vi "Untitled 1.vi"() -> ()   [LabVIEW 2013]
uses:
  <vilib>/Analysis/6fits.llb/General Linear Fit Algorithm.ctl
  <vilib>/Analysis/NI_AALPro.lvlib
panel:
  in  "algorithm":T1 items=["SVD", "Givens", "Givens2", "Householder", "LU Decomposition", "Cholesky", "SVD for Rank Deficient H"]
  out "residue":dbl
  out "Polynomial Coefficients":dbl[](array[numeric])
  out "Best Polynomial Fit":dbl[](array[numeric])
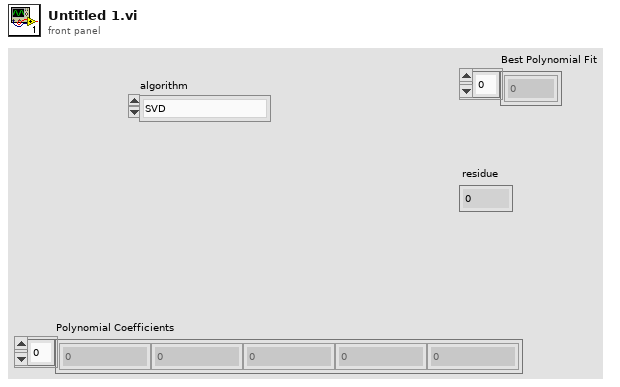
[diagram p1: front panel]
types:
  T1 = typedef "NI_AALPro.lvlib/General Linear Fit Algorithm.ctl" = u16
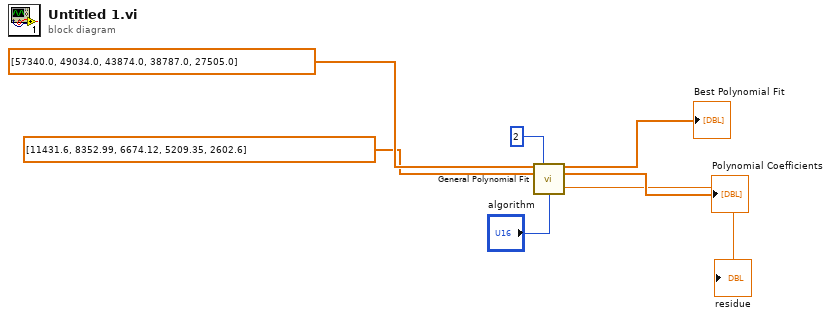
[diagram p0: block diagram]
diagram:
  n1 = call <vilib>:"General Polynomial Fit.vi"("Y"=dbl[] [57340.0, 49034.0, 43874.0, 38787.0, 27505.0], "polynomial order"=2, "X"=dbl[] [11431.6, 8352.99, 6674.12, 5209.35, 2602.6], "algorithm"="algorithm") -> ("Best Polynomial Fit"=→"Best Polynomial Fit":dbl[], "Polynomial Coefficients"=→"Polynomial Coefficients":dbl[], "residue"=→"residue":dbl)  [unwired: 8 in, 1 out]
